vi "RT_SynthFoc_V2_GPU.vi"(0 "Ann Array Params":T1={"Synth Foc?"=FALSE, "Focal Zones"=41, "Switch T/R"=0, "Trans Geometry (mm)"={"Transducer"=0, "Geo Focus"=12.0, "a (radius)"=3.0, "# of rings"=5, "kerf space "=0.1, "Center Freq"=12.0}, "Sub Ap Excite?"=FALSE, "Full Array Scan?"=FALSE, "Xmt/Rcv"={"XMIT"=[TRUE, TRUE, TRUE, TRUE, TRUE], "RCV"=[TRUE, TRUE, TRUE, TRUE, TRUE]}, "PulseSpacing (us)"=0.0, "Xmit Ring"=0, "XMIT CHS"=0, "RCV CHS"=0, "GPU?"=FALSE, "Save TIFF?"=FALSE, "downfactor"=1, "RCV 1CH"=0} {"RCV 1CH" items=["All", "1", "2", "3", "4", "5"]; "Trans Geometry (mm)"."Transducer" items=["6D 12R 40 MHz"=0, "10D 31R 20 MHz"=1, "10D 23R 20 MHz"=2, "6D 23R 40 MHz"=3, "4.5D 10.7R 40 MHz"=4, "9D 23.5R 20 MHz"=5, "9D 25.8R 20MHz"=6, "Enter"=99]; "Switch T/R" min=1 max=5 step=1}, 2 "Pause?":bool, 3 "Motion Settings":T4={"No Motion?"=FALSE, "Motion System"=enum."NI 735x", "Motion Bd ID"=1, "Motion Profile"="SMAC1", "# Axis"=1, "Reverse Z axis?"=TRUE, "SMAC Axis"=0, "scan pair"=enum."y-(x) scan", "RT fps"=6.0, "Steps per mm"=[1000, 1000, 1000, 1000], "Motor Parameters"={"velocity ct/s"=[10000.0, 10000.0, 10000.0, 50000.0], "accel ct/s^2"=[50000.0, 50000.0, 50000.0, 200000.0]}, "One Way Scan"=FALSE, "Reverse One Way Scan"=FALSE, "Global Position (mm)"=[], "Plane"=0, "Distance between\nscan lines (um)"=0.0, "Distance between\nscan planes (um)"=0.0, "number of scan planes"=1, "Total steps in line"=0, "Xtra plane\ndistance  (um)"=100, "Xtra planes "=1, "Add Axis"=FALSE, "overshoot cts"=200, "BKPT Shift"=0, "Scan Start Time (ms)"=0, "ESP VISA"="GPIB::1::INSTR", "3rd Axis"=1, "GL Ref Out"=refnum, "Galil Address"=""} {"3rd Axis" items=["x", "y", "z", "w"]; "Xtra planes" min=1; "Xtra plane\ndistance  (um)" min=0; "Distance between\nscan planes (um)" format="%.2f"; "Distance between\nscan lines (um)" format="%.2f"; "SMAC Axis" items=["None"=0, "Axis 1"=1, "Axis 2"=2, "Axis 3"=3, "Axis 4"=4, "Axis 5"=5, "Axis 6"=6, "Axis 7"=7, "Axis 8"=8, "Vector Space 1"=17, "Vector Space 2"=18, "Vector Space 3"=19, "Vector Space 4"=20]; "Motion Bd ID" min=1 max=32 step=1}, 4 "Scan Axis":i32, 7 "Digitizer Settings":T8={"Digitizer delay (us) "=0.0, "rf points per line"=2048, "lines per plane"=128, "Samp Rate (Hz)"=100000000.0, "Additional dig delay (us)"=0.0, "Voltage Scale"=0.4, "Pre-Looks"=0, "Offset delay (us)"=0.0, "bits A/D"=8, "Avg Num"=1, "DigTimeOut"=5.0, "Rel Dig Delay"=0.0, "Dig Ch"=0, "LeCroyCluster"={"LeCroy Channels"=[TRUE, FALSE, FALSE, FALSE], "LC read pt offset"=0.0, "Sweep Avg"=FALSE}, "Main Digitizer"=enum."NI Digitizer", "Dig Config"=enum."Single channel", "Digitizer ID Cluster"={"Acqiris/Alazar/SP ID"=[], "NI Instr Handles"=[], "LeCroy VISA"="", "GaGe Handle"={"Handle"=0, "Sample size"=0, "Resolution"=0, "Offset"=0, "Channels"=0, "Boards"=0}, "ATS Ref"="ATS9350", "Acqiris Address"=["PCI::INSTR0"], "ADQRef"=refnum, "adq_cu_ptr"=refnum}, "Trigger Settings"={"Trig Source"=1, "Trig Coupling"=0, "Trig Slope"=0, "Level (mV)"=1500.0}, "Bulk Acq"=FALSE, "Bulk Start Indexes"=[], "Data Ref RF"=refnum, "NI ID/Channel"=[], "Total Dig CH"=1, "Xtra Ann Trig delay (us)"=10.0, "Fix Z Delay?"=FALSE, "One Way Transmission?"=FALSE, "Data Ref Log"=refnum} {"Trigger Settings"."Trig Slope" items=["Positive", "Negative"]; "Trigger Settings"."Level (mV)" format="%.2f"; "Trigger Settings"."Trig Coupling" items=["DC 1 MOhm", "AC 1 MOhm", "DC 50 Ohm", "AC 50 Ohm"]; "Trigger Settings"."Trig Source" items=["Chan 1", "External"]; "Rel Dig Delay" format="%.2f"; "DigTimeOut" format="%.2f"; "Avg Num" min=1; "Offset delay (us)" format="%.2f"; "Additional dig delay (us)" format="%.2f"; "Digitizer delay (us)" format="%.2f"}, 9 "Qs and Notis":T12, 11 "Raw Name":string="raw") -> (16 "Bd ID Out":u8, 19 "error out":errorcluster)   [LabVIEW 2022 SP3]
uses:
  <vilib>/picture/picture.llb/imagedata.ctl
  ScanningControl/Digitizers/-DigitizerRoutines/DigitizerSettings.ctl
  ScanningControl/Digitizers/-DigitizerRoutines/Digitizer.ctl
  ScanningControl/Digitizers/-DigitizerRoutines/DigConfig.ctl
  ScanningControl/Digitizers/-DigitizerRoutines/DigitizerID.ctl
  C:/Windows/System32/ADQAPI_dotNet_helper.dll
  Windows/System32/ADQAPI_dotNet_helper.dll
  ScanningControl/Motion Controllers/NI_controller/-NI_MotionRoutines/MotionParameters.ctl
  ScanningControl/Motion Controllers/NI_controller/-NI_MotionRoutines/MotionSys.ctl
  ScanningControl/Motion Controllers/-MotionRoutines/ScanAxis.ctl
  ScanningControl/Motion Controllers/-MotionRoutines/3rdAxis.ctl
  Annular Array/-AnnularRoutines/AnnularArray.ctl
  Annular Array/-AnnularRoutines/TransGeometry.ctl
  Annular Array/-AnnularRoutines/ArrayGeometry.ctl
  ScanningControl/Motion Controllers/Galil/Command Menu.ctl
  <vilib>/DAQmx/write.llb/DAQmx Write (Digital Bool 1Line 1Point).vi
  <instrlib>/niScope/Acquire/niScope Get Scaling Coefficients.vi
  ScanningControl/Motion Controllers/-MotionRoutines/MotionGlobals.vi
  <vilib>/DAQmx/miscellaneous.llb/DAQmx Fill In Error Info.vi
  <instrlib>/niScope/Acquire/Fetch/niScope Multi Fetch Binary 8.vi
  <vilib>/Motion/FlexMotion/FunctionsVIs/Trajectory.llb/Load Acceleration/Deceleration.flx
  <vilib>/Motion/FlexMotion/CustomControls/CustomControls.llb/Program.flx
  <vilib>/Motion/FlexMotion/FunctionsVIs/Trajectory.llb/Wait for Move Complete (8 axes).flx
  <vilib>/Analysis/NI_AALPro.lvlib
  <instrlib>/LeCroy Wave Series/LeCroy Wave Series.lvlib
panel:
  in  "Round to ROC?":bool
  in  "One Way Receive":bool
  # "1-D and 2-D B scan settings"
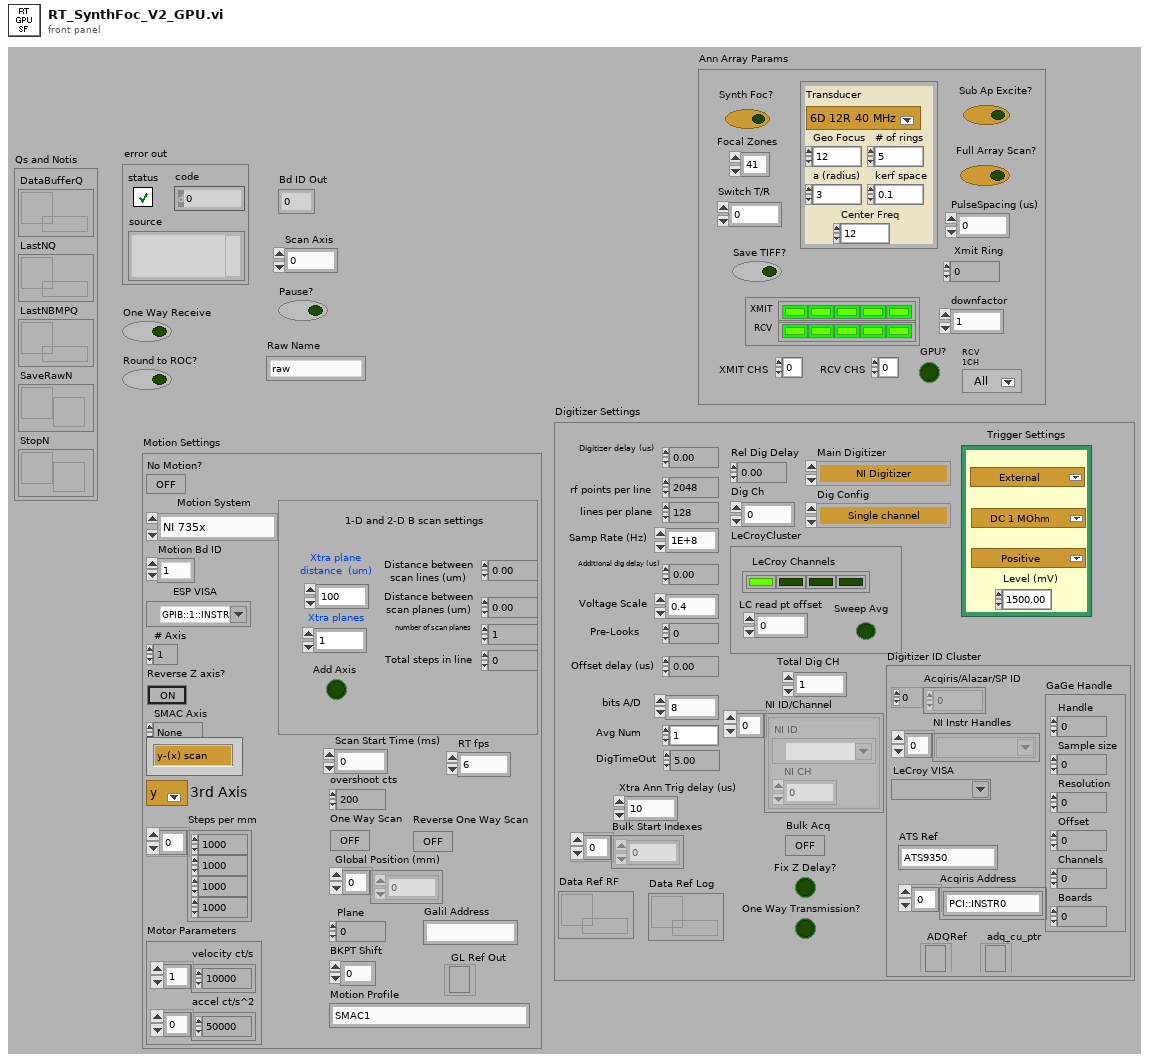
[diagram p1: front panel]
types:
  T1 = typedef "AnnularArray.ctl" = cluster{"Synth Foc?":bool, "Focal Zones":i16, "Switch T/R":i16, "Trans Geometry (mm)":T2, "Sub Ap Excite?":bool, "Full Array Scan?":bool, "Xmt/Rcv":cluster{"XMIT":bool[], "RCV":bool[]}, "PulseSpacing (us)":sgl, "Xmit Ring":i32, "XMIT CHS":u8, "RCV CHS":u8, "GPU?":bool, "Save TIFF?":bool, "downfactor":i32, "RCV 1CH":u16}
  T2 = typedef "TransGeometry.ctl" = cluster{"Transducer":T3, "Geo Focus":dbl, "a (radius)":dbl, "# of rings":i32, "kerf space ":dbl, "Center Freq":dbl}
  T3 = typedef "ArrayGeometry.ctl" = u16
  T4 = typedef "MotionParameters.ctl" = cluster{"No Motion?":bool, "Motion System":T5, "Motion Bd ID":u8, "Motion Profile":string, "# Axis":i8, "Reverse Z axis?":bool, "SMAC Axis":u16, "scan pair":T6, "RT fps":sgl, "Steps per mm":i32[], "Motor Parameters":cluster{"velocity ct/s":dbl[], "accel ct/s^2":dbl[]}, "One Way Scan":bool, "Reverse One Way Scan":bool, "Global Position (mm)":dbl[], "Plane":i32, "Distance between\nscan lines (um)":sgl, "Distance between\nscan planes (um)":sgl, "number of scan planes":i32, "Total steps in line":i32, "Xtra plane\ndistance  (um)":i32, "Xtra planes ":i32, "Add Axis":bool, "overshoot cts":i32, "BKPT Shift":i32, "Scan Start Time (ms)":u32, "ESP VISA":refnum<visa-resource-name>, "3rd Axis":T7, "GL Ref Out":refnum<k7>, "Galil Address":string}
  T5 = typedef "MotionSys.ctl" = enum16{"MM3000", "NI 735x", "Newport ESP", "No Motion Card", "Galil"}
  T6 = typedef "ScanAxis.ctl" = enum16{"y-(x) scan", "x-(y) scan", "z-(x) scan", "z-(y) scan", "y-(z) scan", "x-(z) scan", "w-(x) scan", "w-(y) scan", "w-(z) scan", "x-(w) scan", "y-(w) scan", "z-(w) scan"}
  T7 = typedef "3rdAxis.ctl" = u16
  T8 = typedef "DigitizerSettings.ctl" = cluster{"Digitizer delay (us) ":dbl, "rf points per line":i32, "lines per plane":i32, "Samp Rate (Hz)":dbl, "Additional dig delay (us)":dbl, "Voltage Scale":dbl, "Pre-Looks":i32, "Offset delay (us)":dbl, "bits A/D":i8, "Avg Num":i32, "DigTimeOut":sgl, "Rel Dig Delay":sgl, "Dig Ch":i32, "LeCroyCluster":cluster{"LeCroy Channels":bool[], "LC read pt offset":dbl, "Sweep Avg":bool}, "Main Digitizer":T9, "Dig Config":T10, "Digitizer ID Cluster":T11, "Trigger Settings":cluster{"Trig Source":u16, "Trig Coupling":u16, "Trig Slope":u16, "Level (mV)":dbl}, "Bulk Acq":bool, "Bulk Start Indexes":i32[], "Data Ref RF":refnum<data-value>, "NI ID/Channel":cluster{"NI ID":refnum<k15>, "NI CH":i32}[], "Total Dig CH":i32, "Xtra Ann Trig delay (us)":dbl, "Fix Z Delay?":bool, "One Way Transmission?":bool, "Data Ref Log":refnum<data-value>}
  T9 = typedef "Digitizer.ctl" = enum16{"Acqiris Digitizer", "NI Digitizer", "LeCroy", "GaGe", "AlazarTech", "No Digitizer", "Teledyne"}
  T10 = typedef "DigConfig.ctl" = enum16{"Single channel", "2 Chans w/ 2 Acqiris", "2 Chans w/ 1 Acqiris", "5-CH Pulser New", "5-CH pulser w/ ann array", "5-pass style ann array", "Empty"}
  T11 = typedef "DigitizerID.ctl" = cluster{"Acqiris/Alazar/SP ID":u32[], "NI Instr Handles":refnum<k15>[], "LeCroy VISA":refnum<visa-resource-name>, "GaGe Handle":cluster{"Handle":u32, "Sample size":u32, "Resolution":i32, "Offset":i32, "Channels":u32, "Boards":u32}, "ATS Ref":string, "Acqiris Address":string[], "ADQRef":refnum<k24>, "adq_cu_ptr":refnum<k24>}
  T12 = cluster{"DataBufferQ":refnum<queue>, "LastNQ":refnum<queue>, "LastNBMPQ":refnum<queue>, "SaveRawN":refnum<notifier>, "StopN":refnum<notifier>}
  T13 = cluster{"offset":dbl, "gain":dbl, "reserved 1":dbl, "reserved 2":dbl}[]
  T14 = cluster{"offset":dbl, "gain":dbl, "reserved 1":dbl, "reserved 2":dbl}
  T15 = cluster{sgl, "Gain [dB]  ":sgl, "Atten (dB)":sgl}
  T16 = typedef "location.ctl" = enum16{"Automatic", "WCM Main", "Hawaii", "Columbia MM3000", "Columbia  NI System", "NYU", "RRI 2", "UHI Allen", "CUMC RT", "Chiba", "Stony Brook", "WCM Microscopy", "WCM Aeoretch", "WCM Optics Lab", "WCM Main 2Axis", "WCM Rotation", "WCM SAM SMAC", "SERI GP"}
  T17 = typedef "Command Menu.ctl" = enum16{"CommandPassThrough", "Abort Motion", "Define Pos", "Velocity", "Acceleration", "Deceleration", "Position Rel", "Postion Abs", "Begin Move", "After Move", "Home", "KI", "KD", "KP", "IL", "Config I/O", "Set Bit", "Clear Bit", "Motor Off", "Moto On", "Status", "Execute", "Halt Execute", "HX Status", "Tell Velocity", "Check Motion", "BreakPoint", "Tell Position", "Current Code Line", "Tell Switches", "OC Force On", "OC Off", "Pos Soft Limit", "Rev Soft Limit"}
  T18 = cluster{"gain":dbl, "wfm":i16[], bool, bool, i32}
  T19 = typedef "Program.flx" = u8
  T20 = cluster{"data value reference":refnum<data-value>, "bytes to transfer":u32, "rf pts actual":u32}
  T21 = cluster{"gain":dbl, bool, "RF_Out":i16[][], "count":i32, bool}
  T22 = cluster{"actualSamples":i32, "absoluteInitialX":dbl, "relativeInitialX":dbl, "xIncrement":dbl, "offset":dbl, "gain":dbl, "reserved1":dbl, "reserved2":dbl}[]
  T23 = cluster{"actualSamples":i32, "absoluteInitialX":dbl, "relativeInitialX":dbl, "xIncrement":dbl, "offset":dbl, "gain":dbl, "reserved1":dbl, "reserved2":dbl}
  T24 = cluster{"gain":dbl, "Sorted Array Out":i16[], "Reverse?":bool, "status":bool, i32}
  T25 = cluster{"Raw VGain (scale)":dbl, "Sorted Array Out":i16[], "Reverse?":bool, "status":bool, i32}
  T26 = cluster{"Voltage Scale":dbl, "DataInterleavedOut":i16[], "Reverse?":bool, bool, i32}
  T27 = typedef "Bd Id Out" = u8
  T28 = typedef "Resource Out (Enum).flx" = u16
  T29 = typedef "GL Axis Control.ctl" = u16
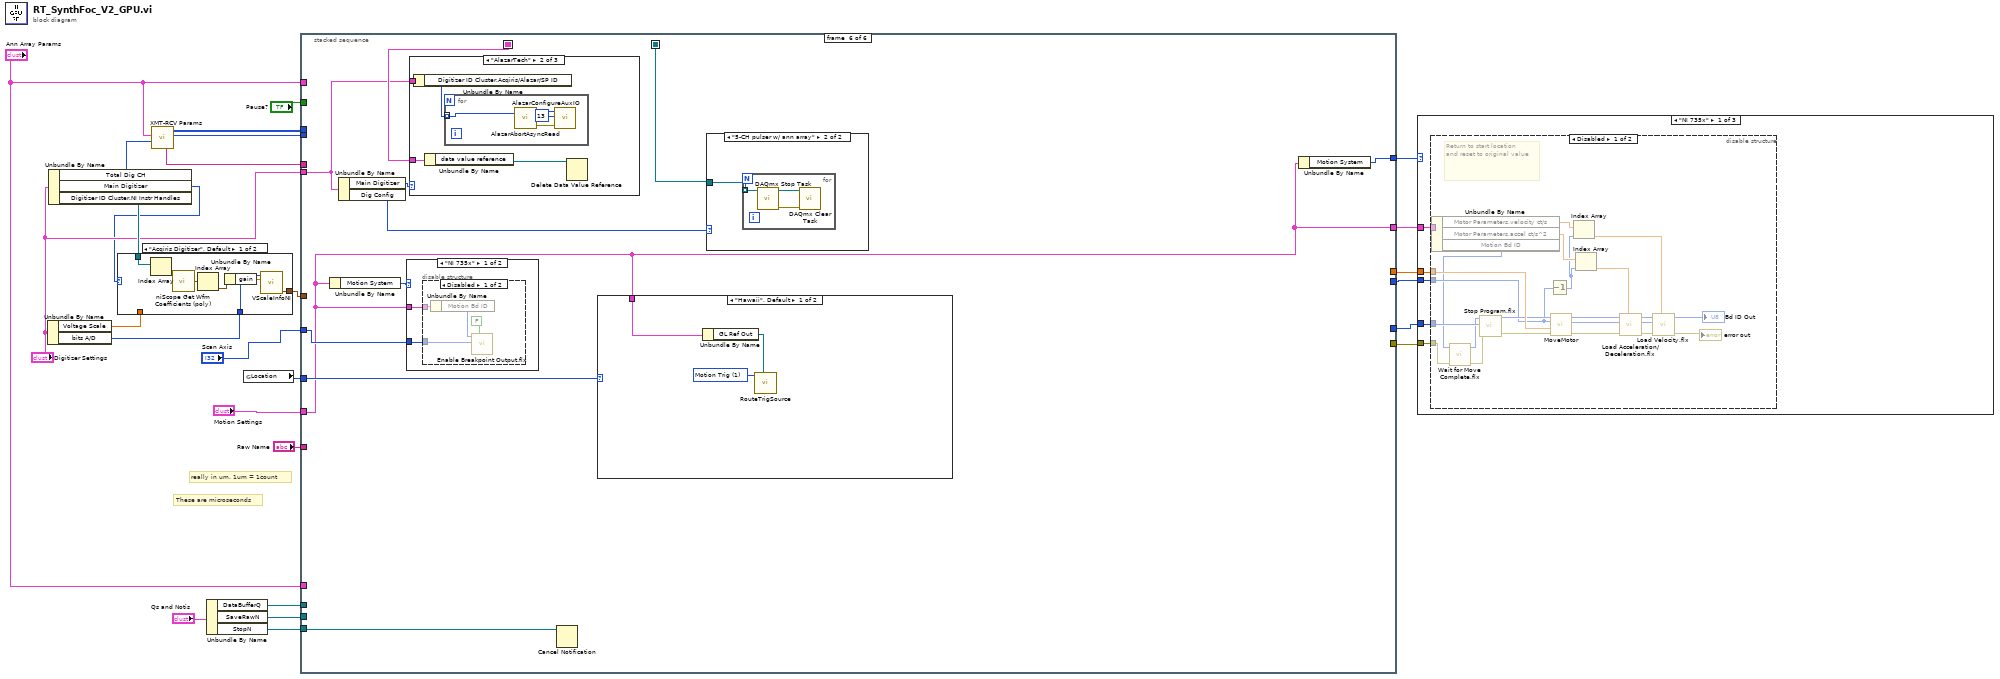
[diagram p0: block diagram]
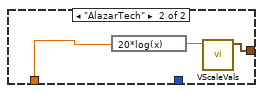
[diagram p2: hidden frame]
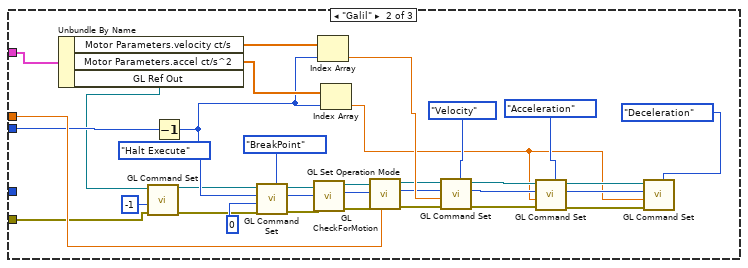
[diagram p4: hidden frame]
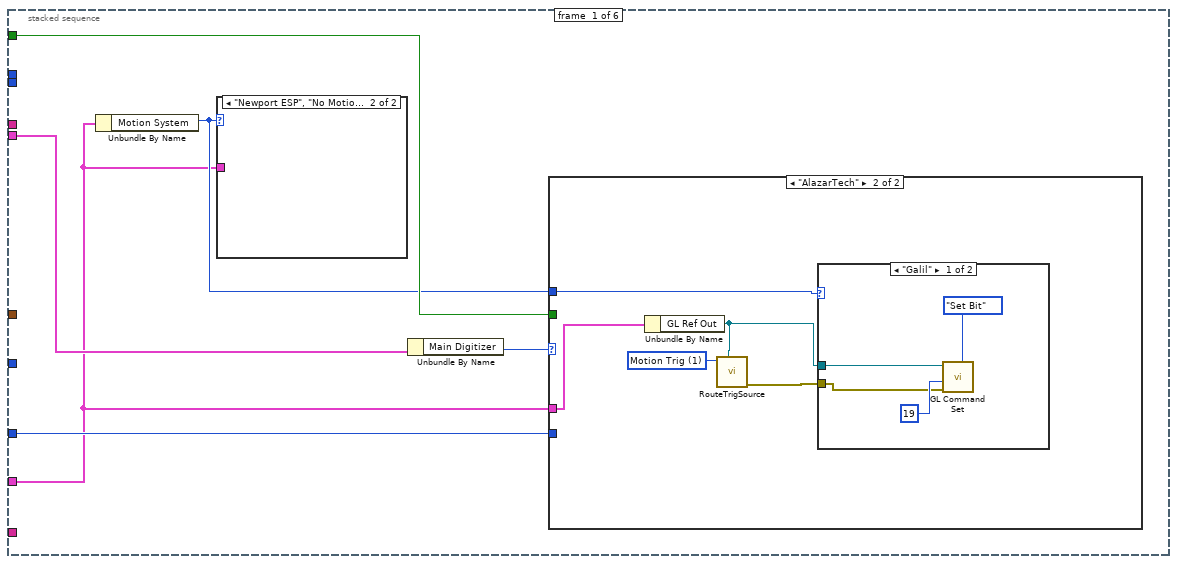
[diagram p6: hidden frame]
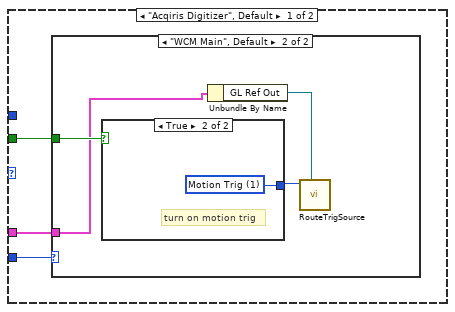
[diagram p7: hidden frame]
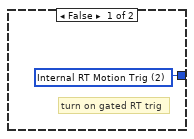
[diagram p9: hidden frame]
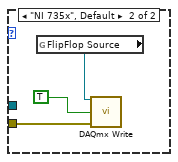
[diagram p10: hidden frame]
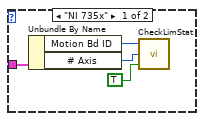
[diagram p11: hidden frame]
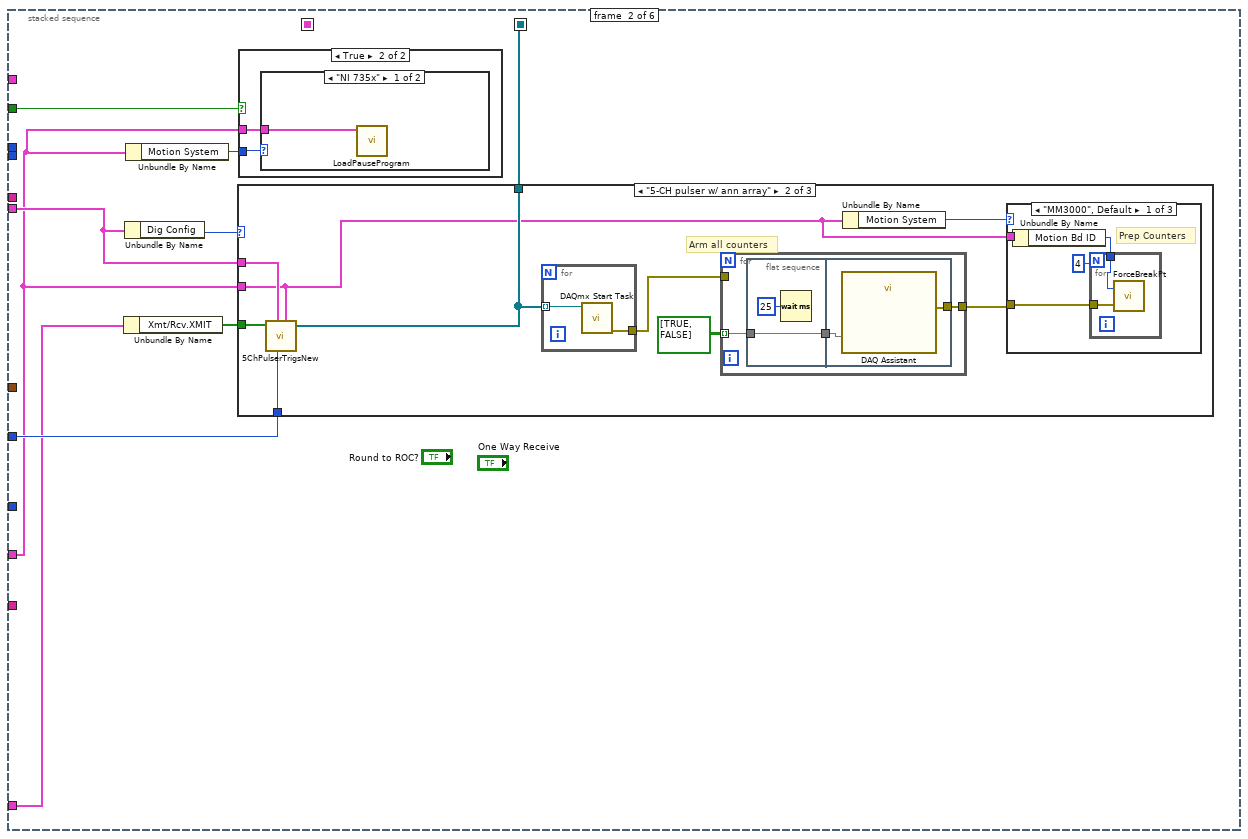
[diagram p12: hidden frame]
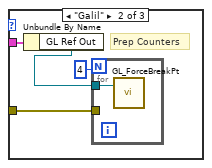
[diagram p14: hidden frame]
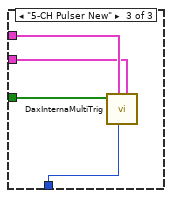
[diagram p16: hidden frame]
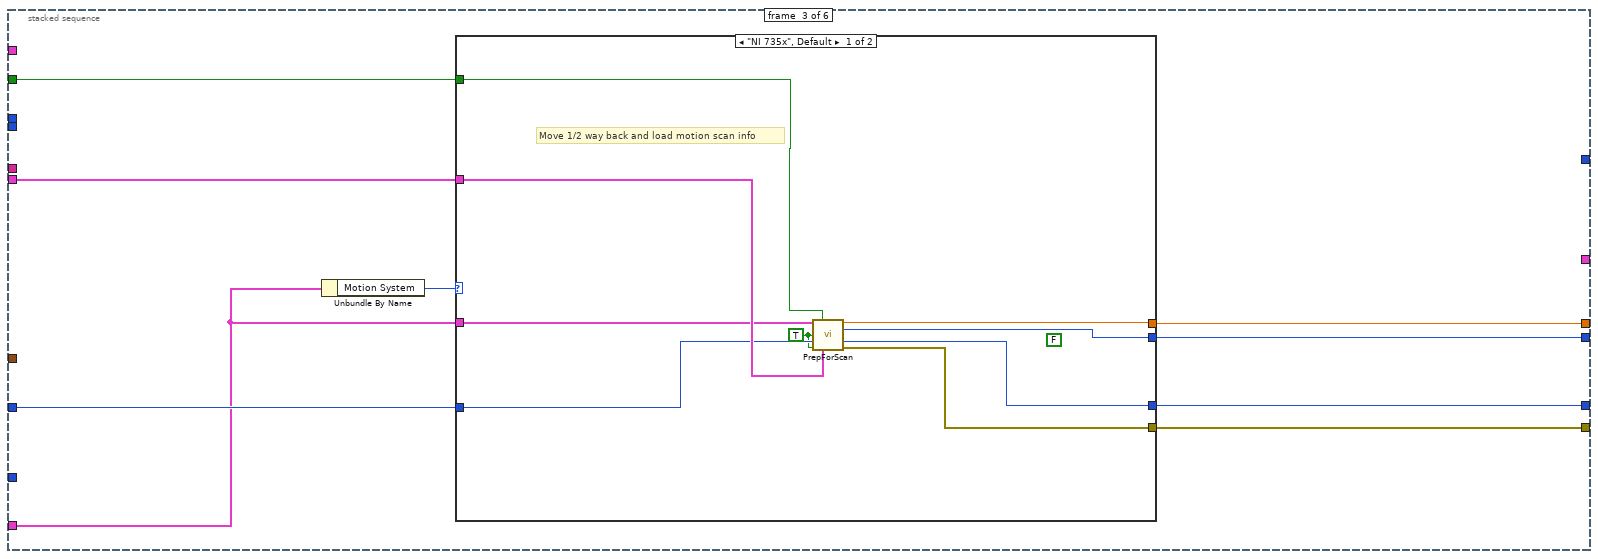
[diagram p19: hidden frame]
diagram:
  # "These are microseconds"
  # "really in um. 1um = 1count"
  n1 = Unbundle By Name("Digitizer Settings") -> ("Voltage Scale"=w11:dbl, "bits A/D"=w10:i8)
  n2 = Unbundle By Name("Digitizer Settings") -> ("Total Dig CH"=w2:i32, "Main Digitizer"=w8:T9, "Digitizer ID Cluster.NI Instr Handles"=w12:refnum<k15>[])
  n3 = case shown="\"Acqiris Digitizer\", Default" w8 {
    tunnel: [w29 w35] -> w15
    tunnel: w12 -> [w28 _]
    tunnel: w10 -> [w27 _]
    tunnel: w11 -> [_ w34]
    frame "Acqiris Digitizer", Default {
      n4 = Index Array(array=w28) -> (element=w31:refnum<k15>)  [unwired: 1 in]
      n5 = call-poly <instrlib>:"niScope Get Wfm Coefficients (poly).vi"("instrument handle"=w31) -> ("coefficient info"=w32:T13)  [unwired: 12 in, 2 out]
      n6 = Index Array(array=w32) -> (element=w33:T14)  [unwired: 1 in]
      n7 = Unbundle By Name(w33) -> ("gain"=w30:dbl)
      n8 = call "VScaleInfoNI.vi"("A/D bits"=w27, "gain"=w30) -> ("Voltage Scale"=w29:T15)  [unwired: 5 in, 3 out]
    }
    frame "AlazarTech" {
      n9 = expression code="20*log(x)"(w34) -> (w36:dbl)
      n10 = call "VScaleVals.vi"("Full Scale"=w36) -> ("Voltage Scale"=w35:T15)  [unwired: 8 in, 2 out]
    }
  }
  n11 = call "XMT-RCV Params.vi"("Dig Channels"=w2, "Ann Array Params"="Ann Array Params") -> ("# XMIT"=w14:i16, "Recip Table"=w13:i16[][], "T/R String"=w7:string)  [unwired: 4 in, 3 out]
  n12 = Unbundle By Name("Qs and Notis") -> ("DataBufferQ"=w20:refnum<queue>, "SaveRawN"=w19:refnum<notifier>, "StopN"=w21:refnum<notifier>)
  n13 = global read "MotionGlobals.vi" "Location"() -> (w16:T16)
  n14 = stacked-sequence {
    seq-local: [_ w75 _ _ _ _] -> [_ _ _ _ _ w552]
    seq-local: [_ _ _ w135 _ _] -> [_ _ _ _ w192 w548]
    tunnel: [_ _ w121 _ _ _] -> w24
    tunnel: [_ _ w120 _ _ _] -> w25
    tunnel: [_ _ w117 _ _ _] -> w23
    tunnel: [_ _ w119 _ _ _] -> w26
    tunnel: "Scan Axis" -> [_ w74 w118 _ _ w549]
    tunnel: w21 -> [_ _ _ _ w216 w550]
    tunnel: w20 -> [_ _ _ _ w205 _]
    tunnel: w16 -> [w42 _ _ _ _ w551]
    tunnel: "Pause?" -> [w41 w76 w116 _ w215 _]
    tunnel: w19 -> [_ _ _ _ w214 _]
    tunnel: "Raw Name" -> [_ _ _ _ w213 _]
    tunnel: w15 -> [_ _ _ _ w211 _]
    tunnel: w14 -> [_ _ _ w137 w210 _]
    tunnel: w13 -> [_ _ _ _ w188 _]
    tunnel: w7 -> [_ _ _ _ w209 _]
    tunnel: "Digitizer Settings" -> [w39 w72 w115 w132 w185 w547]
    tunnel: "Motion Settings" -> [w37 w68 w114 _ w197 w542]
    tunnel: [_ _ _ _ _ w543] -> w6
    tunnel: [_ _ _ _ _ w542] -> w5
    tunnel: "Ann Array Params" -> [_ w69 _ _ w183 _]
    tunnel: "Ann Array Params" -> [_ _ _ _ w187 _]
    frame #0 {
      n15 = Unbundle By Name(w37) -> ("Motion System"=w38:T5)
      n16 = case shown="\"Newport ESP\", \"No Motion Card\", Default" w38 {
        tunnel: w37 -> [w67 _]
        frame "NI 735x" {
          n17 = Unbundle By Name(w67) -> ("Motion Bd ID"=w66:u8, "# Axis"=w65:i8)
          n18 = call "CheckLimStat.vi"("Always Warn?"=TRUE, "# Axis"=w65, "Motion Board ID"=w66) -> ()  [unwired: 3 in]
        }
        frame "Newport ESP", "No Motion Card", Default {
        }
      }
      n19 = Unbundle By Name(w39) -> ("Main Digitizer"=w40:T9)
      n20 = case shown="\"AlazarTech\"" w40 {
        tunnel: w42 -> [w45 _]
        tunnel: w41 -> [w44 _]
        tunnel: w38 -> [_ w54]
        tunnel: w37 -> [w43 w53]
        frame "Acqiris Digitizer", Default {
          n21 = case shown="\"WCM Main\", Default" w45 {
            tunnel: w44 -> [_ w49]
            tunnel: w43 -> [_ w47]
            frame "UHI Allen", "CUMC RT" {
            }
            frame "WCM Main", Default {
              n22 = case shown="True" w49 {
                tunnel: [w50 w51] -> w48
                frame False {
                  w50 = u16 2 items=["Function Gen Input", "Motion Trig", "Internal RT Motion Trig", "Internal CTR 1 Output"] ("Trig Source")
                  # "turn on gated RT trig"
                }
                frame True {
                  w51 = u16 1 items=["Function Gen Input", "Motion Trig", "Internal RT Motion Trig", "Internal CTR 1 Output"] ("Trig Source")
                  # "turn on motion trig"
                }
              }
              n23 = Unbundle By Name(w47) -> ("GL Ref Out"=w46:refnum<k7>)
              n24 = call "RouteTrigSource.vi"("Galil.IGalil"=w46, "Trig Source"=w48) -> ()  [unwired: 9 in, 1 out]
            }
          }
        }
        frame "AlazarTech" {
          w56 = u16 1 items=["Function Gen Input", "Motion Trig", "Internal RT Motion Trig", "Internal CTR 1 Output"] ("Trig Source")
          n25 = Unbundle By Name(w53) -> ("GL Ref Out"=w52:refnum<k7>)
          n26 = call "RouteTrigSource.vi"("Galil.IGalil"=w52, "Trig Source"=w56) -> ("error out"=w55:errorcluster)  [unwired: 9 in]
          n27 = case shown="\"Galil\"" w54 {
            tunnel: w55 -> [w58 w61]
            tunnel: w52 -> [w57 _]
            frame "Galil" {
              n28 = call "GL Command Set.vi"("Command"=Command_Menu."Set Bit", "error in (no error)"=w58, "Value"=19, "Galil.IGalil"=w57) -> ()  [unwired: 3 in, 5 out]
            }
            frame "NI 735x", Default {
              n29 = global read "MotionGlobals.vi" "FlipFlop Source"() -> (w62:refnum<k21>)
              n30 = call-poly <vilib>:"DAQmx Write.vi"("task/channels in"=w62, "data"=TRUE ("stop (T)"), "error in"=w61) -> ()  [unwired: 10 in, 3 out]
            }
          }
        }
      }
    }
    frame #1 {
      n31 = Unbundle By Name(w69) -> ("Xmt/Rcv.XMIT"=w70:bool[])
      n32 = Unbundle By Name(w72) -> ("Dig Config"=w73:T10)
      n33 = Unbundle By Name(w68) -> ("Motion System"=w71:T5)
      n34 = case shown="\"5-CH pulser w/ ann array\"" w73 {
        tunnel: w74 -> [_ w85 w106]
        tunnel: [_ w84 _] -> w75
        tunnel: w70 -> [_ w80 w107]
        tunnel: w72 -> [_ w79 w109]
        tunnel: w68 -> [_ w77 w108]
        frame "Single channel", Default {
        }
        frame "5-CH pulser w/ ann array" {
          # "Arm all counters"
          n35 = call "5ChPulserTrigsNew.vi"("Motion Settings"=w77, "Digitizer Settings"=w79, "XMIT"=w80, "Axis"=w85) -> ("5CH Pulser Tasks"=w84:refnum<k21>[])  [unwired: 5 in, 1 out]
          n36 = for {
            tunnel: w84 -> [w98] mode=indexing
            tunnel: [w97] -> w82
            n37 = call <vilib>:"DAQmx Start Task.vi"("task/channels in"=w98) -> ("error out"=w97:errorcluster)  [unwired: 1 in, 13 out]
          }
          n38 = for {
            tunnel: bool[][] [[TRUE], [FALSE]] ("data") -> [w100] mode=indexing
            tunnel: w82 -> [_]
            tunnel: [w99] -> w81
            n39 = flat-sequence {
              tunnel: w100 -> [w103]
              tunnel: [w103] -> w101
              tunnel: w101 -> [w105]
              tunnel: [w104] -> w99
              frame #0 {
                n40 = Wait (ms)(milliseconds to wait=u32 25) -> ()  [unwired: 1 out]
              }
              frame #1 {
                n41 = call "DAQ Assistant"("data"=w105) -> ("error out"=w104:errorcluster)  [unwired: 17 in, 1 out]
              }
            }
          }
          n42 = Unbundle By Name(w77) -> ("Motion System"=w78:T5)
          n43 = case shown="\"MM3000\", Default" w78 {
            tunnel: w81 -> [w88 w94 _]
            tunnel: w77 -> [w86 w93 _]
            frame "MM3000", Default {
              # "Prep Counters"
              n44 = Unbundle By Name(w86) -> ("Motion Bd ID"=w87:u8)
              n45 = for {
                N: 4 -> [_]
                tunnel: w88 -> [w91]
                tunnel: w87 -> [w90]
                n46 = call "ForceBreakPt.vi"("error in"=w91, "Bd ID in"=w90) -> ()  [unwired: 2 out]
              }
            }
            frame "Galil" {
              # "Prep Counters"
              n47 = Unbundle By Name(w93) -> ("GL Ref Out"=w92:refnum<k7>)
              n48 = for {
                N: 4 -> [_]
                tunnel: w94 -> [_]
                tunnel: w92 -> [w96]
                n49 = call "GL_ForceBreakPt.vi"("GL Ref Out"=w96) -> ()  [unwired: 1 in, 2 out]
              }
            }
            frame "No Motion Card" {
            }
          }
        }
        frame "5-CH Pulser New" {
          n50 = call "DaxInternaMultiTrig.vi"("Motion Settings"=w108, "Digitizer Settings"=w109, "XMIT"=w107, "Axis"=w106) -> ()  [unwired: 6 in, 1 out]
        }
      }
      n51 = case shown="True" w76 {
        tunnel: w71 -> [_ w111]
        tunnel: w68 -> [_ w110]
        frame False {
        }
        frame True {
          n52 = case shown="\"NI 735x\"" w111 {
            tunnel: w110 -> [w112 _]
            frame "NI 735x" {
              n53 = call "LoadPauseProgram.vi"("Motion Settings"=w112) -> ()  [unwired: 10 in, 1 out]
            }
            frame "No Motion Card", Default {
            }
          }
        }
      }
    }
    frame #2 {
      n54 = Unbundle By Name(w114) -> ("Motion System"=w113:T5)
      n55 = case shown="\"NI 735x\", Default" w113 {
        tunnel: [w127 _] -> w121
        tunnel: [w126 _] -> w120
        tunnel: [w125 _] -> w119
        tunnel: w118 -> [w129 _]
        tunnel: [w128 _] -> w117
        tunnel: w116 -> [w123 _]
        tunnel: w115 -> [w130 _]
        tunnel: w114 -> [w122 _]
        frame "NI 735x", Default {
          w124 = TRUE ("Boolean")
          (unwired) FALSE ("Enable")
          # "Move 1/2 way back and load motion scan info"
          n56 = call "PrepForScan.vi"("Motion Settings In"=w122, "Pause?"=w123, "SMAC?"=w124, "Scan Axis"=w129, "MoveBack?"=w124, "Digitizer Settings"=w130) -> ("Counts"=w128:dbl, "Axis Resource out"=w125:u16, "Program ID"=w126:u8, "error out"=w127:errorcluster)  [unwired: 4 in, 2 out]
        }
        frame "No Motion Card" {
        }
      }
    }
    frame #3 {
      # "Set up sampling rete and delay"
      n57 = Unbundle By Name(w132) -> ("Main Digitizer"=w131:T9, "lines per plane"=w133:i32, "rf points per line"=w134:i32)
      n58 = Multiply(x=w137, y=w133) -> (x*y=w136:i32)
      n59 = case shown="\"AlazarTech\"" w131 {
        tunnel: w134 -> [w141 w154 _]
        tunnel: w136 -> [w140 w153 w169]
        tunnel: [_ w155 _] -> w135
        tunnel: w132 -> [w138 w156 w170]
        frame "Acqiris Digitizer", Default {
          n60 = Unbundle By Name(w138) -> ("Digitizer ID Cluster.NI Instr Handles"=w139:refnum<k15>[])
          n61 = for {
            tunnel: w140 -> [w144]
            tunnel: w141 -> [w148]
            tunnel: w139 -> [w145] mode=indexing
            tunnel: w138 -> [w142]
            n62 = property class="niScope"(reference=w145, "Min Number of Points"=w148, "Number of Records"=w144, "Enable Records > Memory"=TRUE) -> (reference out=w147:refnum<k15>, error out=w146:errorcluster)  [unwired: 1 in]
            n63 = call "NI conSamp.vi"("error in"=w146, "Digitizer Settings"=w142, "InstrumentID"=w147) -> ()  [unwired: 1 in, 2 out]
          }
        }
        frame "AlazarTech" {
          n64 = Unbundle By Name(w156) -> ("Digitizer ID Cluster.GaGe Handle.Boards"=w149:u32, "Digitizer ID Cluster.Acqiris/Alazar/SP ID"=w151:u32[])
          n65 = case shown="2, Default" w149 {
            tunnel: [w158 w159] -> w152
            frame 2, Default {
              w158 = u32 3 items=["A"=1, "B"=2, "A + B"=3, "C"=4, "A + C"=5, "A + B"=6, "D"=8, "A + D"=9, "B + D"=10, "C + D"=12, "A + B + C + D"=15] ("Channel")
            }
            frame 16 {
              w159 = u32 15 items=["A"=1, "B"=2, "A + B"=3, "C"=4, "A + C"=5, "A + B"=6, "D"=8, "A + D"=9, "B + D"=10, "C + D"=12, "A + B + C + D"=15] ("Channel")
            }
          }
          n66 = for {
            tunnel: w152 -> [w168]
            tunnel: [w165] -> w157
            tunnel: w156 -> [w164]
            tunnel: [w163] -> w155
            tunnel: w154 -> [w162]
            tunnel: w153 -> [w161]
            tunnel: w151 -> [w160] mode=indexing
            n67 = call "AlazarAcqPrep - ATS-SDK.vi"("Handle"=w160, "Digitizer Settings"=w164, "Enable Trigger Enable"=TRUE, "Channel"=w168, "BuffCount"=6, "rf points per line"=w162, "rf lines per buffer"=w161) -> ("AlazarCluster"=w163:T20, "error out"=w165:errorcluster)  [unwired: 5 in, 2 out]
          }
          n68 = Index Array(array=w151) -> (element=w150:u32)  [unwired: 1 in]
          n69 = call "AlazarStartCapture.vi"("Handle"=w150, "error in (no error)"=w157) -> ()  [unwired: 3 out]
        }
        frame "LeCroy" {
          w180 = FALSE ("Continuous Acquisition Mode (T: On)")
          w171 = u16 2 items=["RealTime", "RIS", "Sequence", "Roll", "WaveStream"] ("Sample Mode (0: RealTime)")
          n70 = Unbundle By Name(w170) -> ("Digitizer ID Cluster.LeCroy VISA"=w173:refnum<visa-resource-name>, "Digitizer delay (us)"=w172:dbl)
          n71 = call <instrlib>:"Configure Continuous Acquisition.vi"("Auto Trigger Enabled (T: Normal)"=w180, "Continuous Acquisition Mode (T: On)"=w180, "VISA resource name"=w173) -> ("error out"=w181:errorcluster, "VISA resource name out"=w182:refnum<visa-resource-name>)  [unwired: 7 in]
          n72 = expression code="-1E-6*x"(w172) -> (w178:dbl)
          n73 = call <instrlib>:"Configure Sample Mode.vi"("error in (no error)"=w181, "Number of Segments (2)"=w169, "Sample Mode (0: RealTime)"=w171, "VISA resource name"=w182) -> ("error out"=w176:errorcluster, "VISA resource name out"=w177:refnum<visa-resource-name>)  [unwired: 6 in]
          n74 = Number To Exponential String(number=w178) -> (E-format string=w179:string)  [unwired: 3 in]
          n75 = Concatenate Strings("TRDL " ("Write Buffer"), w179) -> (w175:string)
          n76 = call <instrlib>:"Write.vi"("error in (no error)"=w176, "Write Buffer"=w175, "VISA resource name"=w177) -> ()  [unwired: 6 in, 3 out]
        }
      }
    }
    frame #4 {
      n77 = Unbundle By Name(w185) -> ("bits A/D"=w199:i8, "lines per plane"=w200:i32, "rf points per line"=w201:i32)
      n78 = Unbundle By Name(w185) -> ("Total Dig CH"=w196:i32)
      n79 = Multiply(x=w196, y=3) -> (x*y=w195:i32)
      n80 = Unbundle By Name(w192) -> ("rf pts actual"=w191:u32)
      n81 = Multiply(x=w210, y=w200) -> (x*y=w190:i32)
      n82 = Unbundle By Name(w187) -> ("Xmt/Rcv.RCV"=w186:bool[])
      n83 = call "RTHeader.vi"("Comment"=w209, "Digitizer Settings"=w185, "Dig Word Size"=w199, "Ann Array Params"=w183, "Votage scaling"=w211, "Motion Settings"=w197) -> ("Header String Out"=w207:string)  [unwired: 8 in, 1 out]
      n84 = Obtain Queue(max queue size (-1, unlimited)=w195, element data type=T18 {"gain"=0.0, "wfm"=[], TRUE, TRUE, 0}) -> (queue out=w206:refnum<queue>)  [unwired: 3 in, 2 out]
      n85 = Unbundle By Name(w185) -> ("Main Digitizer"=w198:T9)
      n86 = case shown="14" w199 {
        tunnel: [_ u16 3 ("Extra Shift")] -> w202
        frame 0, Default {
        }
        frame 14 {
        }
      }
      n87 = Initialize Array(i16 0, w190, w191) -> (w189:i16[][])
      n88 = Subtract(x=w199, y=w202) -> (x-y=w203:u16)
      n89 = while {
        tunnel: w206 -> [w243]
        tunnel: w201 -> [w242]
        tunnel: [w237] -> w204
        tunnel: w200 -> [w241]
        tunnel: w205 -> [w240]
        tunnel: w207 -> [w239]
        tunnel: w216 -> [w229]
        tunnel: w214 -> [w235]
        tunnel: w213 -> [w234]
        tunnel: w210 -> [w232]
        tunnel: w188 -> [w231]
        tunnel: w203 -> [w230]
        tunnel: w183 -> [w228]
        tunnel: w185 -> [w227]
        tunnel: 1000 ("timeout in ms (-1)") -> [w218]
        i -> [w233]
        stop <- w237 stop-if-true
        n90 = Dequeue Element(queue=w243, timeout in ms (-1)=w218) -> (element=w222:T18)  [unwired: 1 in, 3 out]
        n91 = Unbundle(w222) -> (w219:bool)  [unwired: 4 out]
        n92 = case shown="False" w219 {
          tunnel: w241 -> [_ _]
          tunnel: w242 -> [_ _]
          tunnel: [w263 _] -> w221
          tunnel: w239 -> [w262 _]
          tunnel: w222 -> [w261 _]
          tunnel: w235 -> [w259 _]
          tunnel: w234 -> [w258 _]
          tunnel: w233 -> [w257 _]
          tunnel: [w256 _] -> w220
          tunnel: w232 -> [_ _]
          tunnel: w231 -> [_ _]
          tunnel: w230 -> [w255 _]
          tunnel: w228 -> [w254 _]
          tunnel: w227 -> [w249 _]
          tunnel: [w246 _] -> w226
          tunnel: [w245 _] -> w224
          frame False {
            n93 = Unbundle(w261) -> ("gain"=w263:dbl, "wfm"=w253:i16[], w256:bool, w244:i32)  [unwired: 1 out]
            n94 = Get Notifier Status(notifier=w259) -> (current notification=w260:bool)  [unwired: 1 in, 4 out]
            n95 = Unbundle By Name(w249) -> ("bits A/D"=w248:i8)
            n96 = case shown="True" w260 {
              tunnel: w253 -> [_ w269]
              tunnel: w262 -> [_ w273]
              tunnel: w258 -> [_ w272]
              tunnel: w257 -> [_ w271]
              tunnel: w256 -> [_ _]
              tunnel: w255 -> [_ w270]
              frame False {
              }
              frame True {
                n97 = Build Array(w269) -> (w268:i16[][])
                n98 = call "RawRT_Capture.vi"("A/D bits"=w270, "Raw data"=w268, "File Name In"=w272, "DigCard"=i16 -1, "header"=w273, "Iter"=w271) -> ()  [unwired: 6 in]
              }
            }
            n99 = call "GPU_Process.vi"("DataFlag"=w244, "Ann Array Params"=w254, "Digitizer Settings"=w249, "Raw Data In"=w253) -> ("RF_Out"=w246:i16[][])  [unwired: 5 in, 2 out]
            n100 = Decrement(x=w248) -> (x-1=w250:i8)
            n101 = Power Of 2(x=w250) -> (2^x=w251:dbl)
            n102 = Decrement(x=w251) -> (x-1=w247:dbl)
            n103 = Absolute Value(x=w246) -> (abs(x)=w252:i16[][])
            n104 = for {
              tunnel: w252 -> [w266] mode=indexing
              tunnel: [w265] -> w245 mode=indexing
              tunnel: w247 -> [w264]
              n105 = call <vilib>:"Threshold Detector.vi"("threshold"=w264, "X"=w266) -> ("count"=w265:i32)  [unwired: 1 in, 2 out]
            }
          }
          frame True {
          }
        }
        n106 = Add Array Elements(numeric array=w224) -> (sum=w223:i32)
        n107 = Wait on Notification(notifier=w229, timeout in ms (-1)=5) -> (timed out?=w238:bool)  [unwired: 2 in, 3 out]
        n108 = Not(x=w238) -> (.not. x?=w237:bool)
        n109 = Bundle("gain"=w221, w220, "RF_Out"=w226, "count"=w223, w219) -> (w225:T21)  [unwired: 1 in]
        n110 = Lossy Enqueue Element(queue=w240, element=w225) -> ()  [unwired: 1 in, 4 out]
      }
      n111 = while {
        tunnel: w206 -> [w290]
        tunnel: w201 -> [w289]
        tunnel: [w288] -> w208
        tunnel: w216 -> [w279]
        tunnel: w215 -> [w287]
        tunnel: w186 -> [w286]
        tunnel: w198 -> [w285]
        tunnel: w192 -> [w284]
        tunnel: w190 -> [w283]
        tunnel: w185 -> [w281]
        tunnel: w202 -> [w280]
        tunnel: w185 -> [w277]
        tunnel: w197 -> [w276]
        tunnel: w189 -> [w275]
        tunnel: w183 -> [w274]
        i -> [w282]
        stop <- w278 stop-if-true
        # "Read queue and send to files. About same as reading channel by channel"
        n112 = stacked-sequence {
          seq-local: [w296 _ _ _ _] -> [_ w344 _ _ _]
          seq-local: [_ w338 _ _ _] -> [_ _ _ w486 _]
          tunnel: w290 -> [_ w347 _ _ _]
          tunnel: w289 -> [_ w346 _ _ _]
          tunnel: [_ w345 _ _ _] -> w288
          tunnel: w287 -> [w297 _ _ _ _]
          tunnel: w286 -> [_ w343 _ _ _]
          tunnel: w285 -> [w295 w342 _ w488 _]
          tunnel: w284 -> [_ w341 _ w485 _]
          tunnel: w283 -> [w294 w340 _ _ _]
          tunnel: w282 -> [w293 _ _ _ _]
          tunnel: w281 -> [w292 w339 _ w487 _]
          tunnel: w280 -> [_ w337 _ _ _]
          tunnel: w279 -> [_ _ w482 _ _]
          tunnel: [_ _ w481 _ _] -> w278
          tunnel: w277 -> [_ w336 _ _ _]
          tunnel: w276 -> [w291 w333 _ _ w522]
          tunnel: w275 -> [_ w335 _ _ _]
          tunnel: w274 -> [_ w334 _ _ _]
          frame #0 {
            # "Arm boards"
            n113 = case shown="\"AlazarTech\"" w295 {
              tunnel: w297 -> [w304 w324 w328]
              tunnel: [w303 w322 w327] -> w296
              tunnel: w294 -> [w302 _ w329]
              tunnel: w293 -> [_ _ _]
              tunnel: w292 -> [w298 w326 w331]
              tunnel: w291 -> [w299 w321 w330]
              frame "Acqiris Digitizer", Default {
                n114 = Unbundle By Name(w298) -> ("Digitizer ID Cluster.NI Instr Handles"=w301:refnum<k15>[])
                n115 = Reverse 1D Array(array=w301) -> (reversed array=w300:refnum<k15>[])
                n116 = for {
                  N -> [w309]
                  tunnel: w304 -> [w312]
                  tunnel: [w308] -> w303
                  tunnel: w302 -> [w307]
                  tunnel: w300 -> [w306] mode=indexing
                  tunnel: w299 -> [w305]
                  i -> [w310]
                  n117 = Subtract(x=w309, y=w310) -> (x-y=w311:i32)
                  n118 = case shown="1" w311 {
                    tunnel: [_ w320] -> w308
                    tunnel: w312 -> [_ w319]
                    tunnel: [w313 w318] -> _
                    tunnel: w306 -> [w314 w317]
                    tunnel: w307 -> [_ w316]
                    tunnel: w305 -> [_ w315]
                    frame 0, Default {
                      n119 = call <instrlib>:"niScope Initiate Acquisition.vi"("instrument handle"=w314) -> ("error out"=w313:errorcluster)  [unwired: 2 in, 12 out]
                    }
                    frame 1 {
                      # "Start Move"
                      n120 = call "Rapid Read_NI_Done.vi"("NI Card"=w317, "Motion Settings In"=w315, "records"=w316, "Pause?"=w319) -> ("Reverse?"=w320:bool, "error out"=w318:errorcluster)  [unwired: 10 in]
                    }
                  }
                }
              }
              frame "AlazarTech" {
                n121 = Unbundle By Name(w326) -> ("Digitizer ID Cluster.Acqiris/Alazar/SP ID"=w325:u32[])
                n122 = Index Array(array=w325) -> (element=w323:u32)  [unwired: 1 in]
                n123 = call "Rapid Read_Alazar_Done - ATS-SDK.vi"("Handle"=w323, "Motion Settings"=w321, "Pause?"=w324) -> ("Reverse?"=w322:bool)  [unwired: 10 in, 2 out]
              }
              frame "LeCroy" {
                n124 = Unbundle By Name(w331) -> ("Digitizer ID Cluster.LeCroy VISA"=w332:refnum<visa-resource-name>)
                n125 = call "Rapid Read_LeCroy_Done.vi"("Digitizer ID Cluster.LeCroy VISA"=w332, "Motion Settings In"=w330, "records"=w329, "Pause?"=w328) -> ("Reverse?"=w327:bool)  [unwired: 10 in, 1 out]
              }
            }
          }
          frame #1 {
            # "Read data"
            n126 = case shown="\"LeCroy\"" w342 {
              tunnel: w347 -> [w353 w419 w480]
              tunnel: w346 -> [w365 w429 _]
              tunnel: [w356 w422 w479] -> w345
              tunnel: w344 -> [w364 w428 w478]
              tunnel: w343 -> [w363 w427 _]
              tunnel: w341 -> [_ w413 w470]
              tunnel: w340 -> [w362 w426 _]
              tunnel: w339 -> [w361 _ _]
              tunnel: [_ _ w471] -> w338
              tunnel: w337 -> [_ _ w469]
              tunnel: w336 -> [w351 w417 w466]
              tunnel: w335 -> [_ _ _]
              tunnel: w334 -> [w350 w416 w472]
              tunnel: w333 -> [_ _ _]
              frame "Acqiris Digitizer", Default {
                n127 = Unbundle By Name(w361) -> ("NI ID/Channel"=w360:cluster{"NI ID":refnum<k15>, "NI CH":i32}[])
                n128 = for {
                  tunnel: w365 -> [w377]
                  tunnel: w364 -> [w371]
                  tunnel: w363 -> [w376] mode=indexing
                  tunnel: w362 -> [w375]
                  tunnel: w360 -> [w374] mode=indexing
                  tunnel: [w373] -> w349 mode=concatenating
                  tunnel: [w372] -> w359
                  tunnel: [w371] -> w358
                  tunnel: [w369] -> w357
                  tunnel: [w368] -> w355
                  tunnel: w351 -> [w367]
                  tunnel: w350 -> [w366]
                  i -> [w370]
                  n129 = case shown="True" w376 {
                    tunnel: w377 -> [_ w411]
                    tunnel: [_ w410] -> w372
                    tunnel: w370 -> [_ w404]
                    tunnel: [_ w400] -> w368
                    tunnel: w375 -> [_ w398]
                    tunnel: [FALSE ("status") w396] -> w369
                    tunnel: w374 -> [_ w394]
                    tunnel: [w386 w388] -> w373
                    tunnel: w367 -> [w384 w390]
                    tunnel: w366 -> [w381 w389]
                    frame False {
                      # "insert empty data if no receive channel"
                      n130 = Unbundle By Name(w381) -> ("Xmt/Rcv.XMIT"=w379:bool[])
                      n131 = Unbundle By Name(w384) -> ("rf points per line"=w383:i32, "lines per plane"=w382:i32)
                      n132 = Array Size(array=w379) -> (size(s)=w378:i32)
                      n133 = Compound Arithmetic op=MULTIPLY(w383, w382, w378) -> (w380:i32)
                      n134 = Initialize Array(i16 0, w380) -> (w386:i16[])
                    }
                    frame True {
                      n135 = Unbundle By Name(w394) -> ("NI CH"=w393:i32, "NI ID"=w395:refnum<k15>)
                      n136 = Equal To 0?(x=w404) -> (x = 0?=w403:bool)
                      n137 = property class="niScope"(reference=w395, "Fetch Record Number"=0, "Fetch Number of Records"=w398) -> (reference out=w406:refnum<k15>, error out=w405:errorcluster)  [unwired: 1 in]
                      n138 = Number To Decimal String(number=w393) -> (decimal integer string=w392:string)  [unwired: 1 in]
                      n139 = Select(t=1.0, s=w403, f=0.5) -> (s? t:f=w400:dbl)
                      n140 = call-poly <instrlib>:"niScope Fetch (poly).vi"("timeout"=w400, "error in"=w405, "numSamples"=w411, "channels"=w392, "instrument handle"=w406) -> ("error out"=w397:errorcluster, "wfm"=w391:i8[][], "wfm info"=w409:T22, "instrument handle out"=w399:refnum<k15>)  [unwired: 3 out]
                      n141 = call "DeInterleave.vi"("Digitizer Settings"=w390, "Ann Array Params"=w389, "Data in"=w391) -> ("Sorted Array Out"=w388:i16[])  [unwired: 8 in]
                      n142 = case shown="No Error" w397 {
                        tunnel: w399 -> [_ w412]
                        frame No Error {
                        }
                        frame Error {
                          n143 = call <instrlib>:"niScope Abort.vi"("instrument handle"=w412) -> ()  [unwired: 13 in, 2 out]
                        }
                      }
                      n144 = Index Array(array=w409) -> (element=w408:T23)  [unwired: 1 in]
                      n145 = Unbundle By Name(w397) -> ("status"=w396:bool)
                      n146 = Unbundle By Name(w408) -> ("gain"=w410:dbl)
                    }
                  }
                }
                n147 = expression code="x*1000"(w355) -> (w352:dbl)
                n148 = Bundle("gain"=w359, "Sorted Array Out"=w349, "Reverse?"=w358, "status"=w357, 0) -> (w354:T24)  [unwired: 1 in]
                n149 = Enqueue Element(queue=w353, element=w354, timeout in ms (-1)=w352) -> (queue out=w356:refnum<queue>)  [unwired: 1 in, 2 out]
              }
              frame "LeCroy" {
                n150 = for {
                  tunnel: w429 -> [w441]
                  tunnel: w428 -> [w436]
                  tunnel: w427 -> [w440] mode=indexing
                  tunnel: w426 -> [w439]
                  tunnel: [w438] -> w415 mode=concatenating
                  tunnel: [w437] -> w425
                  tunnel: [w436] -> w424
                  tunnel: [w434] -> w423
                  tunnel: [w433] -> w421
                  tunnel: w417 -> [w432]
                  tunnel: w416 -> [w431]
                  tunnel: w413 -> [w430]
                  i -> [w435]
                  n151 = case shown="True" w440 {
                    tunnel: w441 -> [_ _]
                    tunnel: [_ w453] -> w437
                    tunnel: w435 -> [_ w455]
                    tunnel: [_ w460] -> w433
                    tunnel: w439 -> [_ _]
                    tunnel: [FALSE ("status") FALSE ("status")] -> w434
                    tunnel: [w450 w458] -> w438
                    tunnel: w432 -> [w448 w456]
                    tunnel: w431 -> [w445 w459]
                    tunnel: w430 -> [_ _]
                    frame False {
                      # "insert empty data if no receive channel"
                      n152 = Unbundle By Name(w445) -> ("Xmt/Rcv.XMIT"=w443:bool[])
                      n153 = Unbundle By Name(w448) -> ("rf points per line"=w447:i32, "lines per plane"=w446:i32)
                      n154 = Array Size(array=w443) -> (size(s)=w442:i32)
                      n155 = Compound Arithmetic op=MULTIPLY(w447, w446, w442) -> (w444:i32)
                      n156 = Initialize Array(i16 0, w444) -> (w450:i16[])
                    }
                    frame True {
                      n157 = Equal To 0?(x=w455) -> (x = 0?=w463:bool)
                      n158 = call "GetAcqSeqLeCroy.vi"("Digitizer Settings"=w456, "Source (0: Channel 1)"=w455, "save?"=FALSE) -> ("Raw VGain (scale)"=w453:dbl, "Data Array"=w454:i16[][])  [unwired: 18 in, 5 out]
                      n159 = Select(t=1.0, s=w463, f=0.5) -> (s? t:f=w460:dbl)
                      n160 = call "DeInterleave.vi"("Digitizer Settings"=w456, "Ann Array Params"=w459, "Data in"=w454) -> ("Sorted Array Out"=w458:i16[])  [unwired: 8 in]
                    }
                  }
                }
                n161 = expression code="x*1000"(w421) -> (w418:dbl)
                n162 = Bundle("Raw VGain (scale)"=w425, "Sorted Array Out"=w415, "Reverse?"=w424, "status"=w423, 0) -> (w420:T25)  [unwired: 1 in]
                n163 = Enqueue Element(queue=w419, element=w420, timeout in ms (-1)=w418) -> (queue out=w422:refnum<queue>)  [unwired: 1 in, 2 out]
              }
              frame "AlazarTech" {
                n164 = Bundle By Name(cluster=w466, "DigTimeOut"=400.0 ("time out")) -> (w465:T8)
                n165 = call "AlazarStackChannels1Pass.vi"("AlazarCluster"=w470, "Digitizer Settings"=w465, "Extra Shift"=w469, "Ann Array Params"=w472) -> ("Voltage Scale"=w468:dbl, "Return Code"=w471:u32, "DataInterleavedOut"=w467:i16[])  [unwired: 3 in, 2 out]
                n166 = Equal?(x=w471, y=u32 579) -> (x = y?=w476:bool)
                n167 = Bundle("Voltage Scale"=w468, "DataInterleavedOut"=w467, "Reverse?"=w478, w476, 1) -> (w474:T26)  [unwired: 1 in]
                n168 = Enqueue Element(queue=w480, element=w474, timeout in ms (-1)=20.0 ("time out")) -> (queue out=w479:refnum<queue>)  [unwired: 1 in, 2 out]
              }
            }
          }
          frame #2 {
            n169 = Wait on Notification(notifier=w482, timeout in ms (-1)=5) -> (timed out?=w483:bool)  [unwired: 2 in, 3 out]
            n170 = Not(x=w483) -> (.not. x?=w481:bool)
          }
          frame #3 {
            n171 = case shown="\"AlazarTech\"" w488 {
              tunnel: w485 -> [_ w491]
              tunnel: w487 -> [_ w490]
              tunnel: w486 -> [_ w489]
              frame "Acqiris Digitizer", Default {
              }
              frame "AlazarTech" {
                n172 = case shown="512, Default" w489 {
                  tunnel: w491 -> [_ w505]
                  tunnel: w490 -> [_ w504]
                  frame 0 {
                  }
                  frame 512, Default {
                    w496 = u32 268435538 items=["Data Width"=268435465, "Set/Get Async BuffSize"=268435513, "Set/Get Async Buffcount"=268435520, "Get Data Format"=268435522, "Get Samples Per Timestamp Clock"=268435524, "Get Records Captured"=268435525, "Get Async Buffers Pending"=268435536, "Get Async Buffers Pending Full"=268435537, "Get Async Buffers Pending Empty"=268435538, "ECC Mode"=268435528, "Get Aux Input Level"=268435529, "Get Channels Per Board"=268435568, "Pack Mode"=268435570, "Get FPGA Temperature"=268435584] ("Parameter")
                    w497 = u32 268435537 items=["Data Width"=268435465, "Set/Get Async BuffSize"=268435513, "Set/Get Async Buffcount"=268435520, "Get Data Format"=268435522, "Get Samples Per Timestamp Clock"=268435524, "Get Records Captured"=268435525, "Get Async Buffers Pending"=268435536, "Get Async Buffers Pending Full"=268435537, "Get Async Buffers Pending Empty"=268435538, "ECC Mode"=268435528, "Get Aux Input Level"=268435529, "Get Channels Per Board"=268435568, "Pack Mode"=268435570, "Get FPGA Temperature"=268435584] ("Parameter")
                    w502 = u32 268435536 items=["Data Width"=268435465, "Set/Get Async BuffSize"=268435513, "Set/Get Async Buffcount"=268435520, "Get Data Format"=268435522, "Get Samples Per Timestamp Clock"=268435524, "Get Records Captured"=268435525, "Get Async Buffers Pending"=268435536, "Get Async Buffers Pending Full"=268435537, "Get Async Buffers Pending Empty"=268435538, "ECC Mode"=268435528, "Get Aux Input Level"=268435529, "Get Channels Per Board"=268435568, "Pack Mode"=268435570, "Get FPGA Temperature"=268435584] ("Parameter")
                    n173 = Unbundle By Name(w504) -> ("Digitizer ID Cluster.Acqiris/Alazar/SP ID"=w503:u32[])
                    n174 = Index Array(array=w503) -> (element=w495:u32)  [unwired: 1 in]
                    n175 = call "AlazarGetParameter.vi"("Parameter"=w502, "Handle"=w495) -> ("error out"=w499:errorcluster, "Handle"=w501:u64)  [unwired: 2 in, 2 out]
                    n176 = call "AlazarGetParameter.vi"("error in (no error)"=w499, "Parameter"=w496, "Handle"=w501) -> ("error out"=w498:errorcluster, "Handle"=w500:u64)  [unwired: 1 in, 2 out]
                    n177 = call "AlazarGetParameter.vi"("error in (no error)"=w498, "Parameter"=w497, "Handle"=w500) -> ("error out"=w494:errorcluster, "Value"=w492:i32, "Handle"=w493:u64)  [unwired: 1 in, 1 out]
                    n178 = case shown="2, Default" w492 {
                      selector: w492 -> [_ w510]
                      tunnel: w505 -> [_ w512]
                      tunnel: w494 -> [_ w507]
                      tunnel: w493 -> [_ w506]
                      frame 0, 1 {
                      }
                      frame 2, Default {
                        # "Delete surplus buffers"
                        n179 = Decrement(x=w510) -> (x-1=w508:i32)
                        n180 = Unbundle(w512) -> ("data value reference"=w511:refnum<data-value>)  [unwired: 2 out]
                        n181 = for {
                          N: w508 -> [_]
                          tunnel: w511 -> [w515]
                          tunnel: u32 1 ("uTimeout_ms") -> [w516]
                          tunnel: w507 -> [w514]
                          tunnel: w506 -> [w513]
                          n182 = in-place {
                            in-place-border: w516 -> [w521]
                            in-place-border: w514 -> [w518]
                            in-place-border: w513 -> [w517]
                            n183 = in-place-dvr #1(w515) -> (w520:u16[])  [unwired: 1 out]
                            n184 = call "AlazarWaitNextAsyncBufferCompleteU16.vi"("error in (no error)"=w518, "Timeout (ms)"=w521, "Buffer"=w520, "Handle"=w517) -> ("Buffer"=w519:u16[])  [unwired: 3 out]
                            n185 = in-place-dvr #1(w519) -> ()  [unwired: 2 out]
                          }
                        }
                      }
                    }
                  }
                }
              }
            }
          }
          frame #4 {
            # "Check if motion program is paused at end of run. Rare case of done may come up."
            n186 = case shown="4" 0 {
              tunnel: w522 -> [_ w526]
              frame 0, Default {
              }
              frame 4 {
                n187 = Unbundle By Name(w526) -> ("Motion Bd ID"=w525:u8, "Motion System"=w524:T5)
                n188 = case shown="\"NI 735x\"" w524 {
                  tunnel: w525 -> [_ w527]
                  frame "MM3000", Default {
                  }
                  frame "NI 735x" {
                    n189 = disable-structure shown="Disabled" {
                      disable-tunnel: w527 -> [w528 _]
                      frame Disabled {
                        n190 = while {
                          tunnel: [w540] -> _
                          tunnel: [w536] -> _
                          tunnel: enum16{"Done", "Playing", "Paused", "Storing"}."Paused" ("Program Status") -> [w539]
                          tunnel: w528 -> [w538]
                          tunnel: [w532] -> _
                          tunnel: [30 ("DeviceIn")] -> w529
                          i -> [w532]
                          stop <- w533 stop-if-true
                          n191 = call <vilib>:"Read Program Status.flx"("Program (1)"=T19 8, "Board Id"=w538) -> ("error out"=w536:errorcluster, "Bd Id Out"=w540:T27, "Program Status"=w537:enum16{"Done", "Playing", "Paused", "Storing"})  [unwired: 4 in, 1 out]
                          n192 = Unbundle(w536) -> ("status"=w535:bool)  [unwired: 2 out]
                          n193 = Equal?(x=w539, y=w537) -> (x = y?=w534:bool)
                          n194 = Or(x=w534, y=w535) -> (x .or. y?=w533:bool)
                        }
                        n195 = Wait (ms)(milliseconds to wait=w529) -> ()  [unwired: 1 out]
                      }
                      frame Enabled {
                      }
                    }
                  }
                }
              }
            }
          }
        }
      }
      n196 = Release Queue(queue=w208, force destroy? (F)=w204) -> ()  [unwired: 1 in, 3 out]
    }
    frame #5 {
      n197 = Unbundle By Name(w542) -> ("Motion System"=w544:T5)
      n198 = Unbundle By Name(w547) -> ("Main Digitizer"=w546:T9, "Dig Config"=w545:T10)
      n199 = case shown="\"NI 735x\"" w544 {
        tunnel: w549 -> [w554 _]
        tunnel: w542 -> [w553 _]
        frame "NI 735x" {
          n200 = disable-structure shown="Disabled" {
            disable-tunnel: w554 -> [w557 _]
            disable-tunnel: w553 -> [w556 _]
            frame Disabled {
              n201 = Unbundle By Name(w556) -> ("Motion Bd ID"=w555:u8)
              n202 = call <vilib>:"Enable Breakpoint Output.flx"("Enable Breakpoint"=FALSE, "Axis or Encoder"=w557, "Board ID"=w555) -> ()  [unwired: 1 in, 6 out]
            }
            frame Enabled {
            }
          }
        }
        frame "No Motion Card", Default {
        }
      }
      n203 = case shown="\"AlazarTech\"" w546 {
        tunnel: w547 -> [w560 w565 _]
        tunnel: w548 -> [_ w563 _]
        frame "Acqiris Digitizer" {
          n204 = Unbundle By Name(w560) -> ("Digitizer ID Cluster.NI Instr Handles"=w559:refnum<k15>[])
          n205 = for {
            tunnel: w559 -> [w561] mode=indexing
            n206 = call <instrlib>:"niScope Abort.vi"("instrument handle"=w561) -> ()  [unwired: 13 in, 2 out]
          }
        }
        frame "AlazarTech" {
          n207 = Unbundle By Name(w565) -> ("Digitizer ID Cluster.Acqiris/Alazar/SP ID"=w564:u32[])
          n208 = Unbundle By Name(w563) -> ("data value reference"=w562:refnum<data-value>)
          n209 = for {
            tunnel: w564 -> [w567] mode=indexing
            n210 = call "AlazarAbortAsyncRead.vi"("Handle"=w567) -> ("Handle"=w569:u64, "error out"=w568:errorcluster)  [unwired: 1 in, 1 out]
            n211 = call "AlazarConfigureAuxIO.vi"("error in (no error)"=w568, "Mode"=u32 13, "Handle"=w569) -> ()  [unwired: 1 in, 3 out]
          }
          n212 = Delete Data Value Reference(data value reference=w562) -> ()  [unwired: 1 in, 2 out]
        }
        frame "LeCroy", Default {
        }
      }
      n213 = Cancel Notification(0:w550) -> ()  [unwired: 1 in, 3 out]
      n214 = case shown="\"Hawaii\", Default" w551 {
        tunnel: w542 -> [w575 _]
        frame "Hawaii", Default {
          w576 = u16 1 items=["Function Gen Input", "Motion Trig", "Internal RT Motion Trig", "Internal CTR 1 Output"] ("Trig Source")
          n215 = Unbundle By Name(w575) -> ("GL Ref Out"=w574:refnum<k7>)
          n216 = call "RouteTrigSource.vi"("Galil.IGalil"=w574, "Trig Source"=w576) -> ()  [unwired: 9 in, 1 out]
        }
        frame "UHI Allen", "CUMC RT" {
        }
      }
      n217 = case shown="\"5-CH pulser w/ ann array\"" w545 {
        tunnel: w552 -> [_ w570]
        frame "Single channel", Default {
        }
        frame "5-CH pulser w/ ann array" {
          n218 = for {
            tunnel: w570 -> [w573] mode=indexing
            n219 = call <vilib>:"DAQmx Stop Task.vi"("task/channels in"=w573) -> ("task out"=w572:refnum<k21>, "error out"=w571:errorcluster)  [unwired: 13 in]
            n220 = call <vilib>:"DAQmx Clear Task.vi"("task in"=w572, "error in"=w571) -> ()  [unwired: 13 in, 1 out]
          }
        }
      }
      n221 = Unbundle By Name(w542) -> ("Motion System"=w543:T5)
    }
  }
  n222 = case shown="\"NI 735x\"" w6 {
    tunnel: w26 -> [w578 w611 _]
    tunnel: w25 -> [w581 _ _]
    tunnel: w24 -> [w580 w605 _]
    tunnel: w23 -> [w579 w612 _]
    tunnel: w5 -> [w577 w613 _]
    frame "NI 735x" {
      n223 = disable-structure shown="Disabled" {
        disable-tunnel: w581 -> [w604 _]
        disable-tunnel: w580 -> [w603 _]
        disable-tunnel: w579 -> [w602 _]
        disable-tunnel: w578 -> [w587 _]
        disable-tunnel: w577 -> [w583 _]
        frame Disabled {
          # "Return to start location and reset to original value"
          n224 = Unbundle By Name(w583) -> ("Motor Parameters.velocity ct/s"=w589:dbl[], "Motor Parameters.accel ct/s^2"=w588:dbl[], "Motion Bd ID"=w582:u8)
          n225 = call-poly <vilib>:"Wait for Move Complete.flx"("error in (no error)"=w603, "Board ID"=w582) -> ("error out"=w590:errorcluster, "Bd ID Out"=w591:T27)  [unwired: 6 in, 2 out]
          n226 = call <vilib>:"Stop Program.flx"("error in (no error)"=w590, "Program (1)"=w604, "Board ID"=w591) -> ("error out"=w599:errorcluster, "Bd ID Out"=w600:T27)  [unwired: 4 out]
          n227 = Decrement(x=w587) -> (x-1=w586:u16)
          n228 = call "MoveMotor.vi"("error in (no error)"=w599, "Target Position (0)"=w602, "Axis or Vector Space"=w587, "Motion Bd ID"=w600) -> ("error out"=w593:errorcluster, "Resource Output"=w592:u16, "Bd ID Out"=w594:u8)  [unwired: 5 in]
          n229 = Index Array(array=w589, index=w586) -> (element=w585:dbl)
          n230 = Index Array(array=w588, index=w586) -> (element=w584:dbl)
          n231 = call "Load Acceleration/Deceleration.flx"("Acceleration (100000)"=w584, "error in (no error)"=w593, "Axis or Vector Space"=w592, "Board ID"=w594) -> ("error out"=w597:errorcluster, "Resource Output"=w595:T28, "Bd ID Out"=w596:T27)  [unwired: 1 in, 2 out]
          n232 = call <vilib>:"Load Velocity.flx"("Velocity (10000)"=w585, "error in (no error)"=w597, "Axis or Vector Space"=w595, "Board ID"=w596) -> ("error out"=→"error out":errorcluster, "Bd ID Out"=→"Bd ID Out":T27)  [unwired: 4 out]
        }
        frame Enabled {
        }
      }
    }
    frame "Galil" {
      (unwired) Command_Menu."Halt Execute" ("Command")
      n233 = Unbundle By Name(w613) -> ("Motor Parameters.velocity ct/s"=w637:dbl[], "Motor Parameters.accel ct/s^2"=w636:dbl[], "GL Ref Out"=w606:refnum<k7>)
      n234 = call "GL Command Set.vi"("error in (no error)"=w605, "Value"=-1, "Galil.IGalil"=w606) -> ("error out"=w608:errorcluster, "ref out"=w607:refnum<k7>)  [unwired: 4 in, 3 out]
      n235 = Decrement(x=w611) -> (x-1=w617:u16)
      n236 = call "GL Command Set.vi"("Command"=Command_Menu."BreakPoint", "error in (no error)"=w608, "Value"=0, "Axis"=w617, "Galil.IGalil"=w607) -> ("error out"=w622:errorcluster, "Axis Out"=w618:T29, "ref out"=w623:refnum<k7>)  [unwired: 2 in, 2 out]
      n237 = call "GL CheckForMotion.vi"("error in"=w622, "Axis"=w618, "Refnum in"=w623) -> ("error out"=w620:errorcluster, "Axis out"=w619:T29, "Refnum out"=w621:refnum<k7>)  [unwired: 6 in]
      n238 = Index Array(array=w637, index=w617) -> (element=w627:dbl)
      n239 = Index Array(array=w636, index=w617) -> (element=w626:dbl)
      n240 = call "GL Set Operation Mode.vi"("position cts (abs/rel)"=w612, "error in (no error)"=w620, "Axis"=w619, "Galil.IGalil"=w621) -> ("error out"=w614:errorcluster, "Axis Out Output"=w625:T29, "Galil Out"=w624:refnum<k7>)  [unwired: 5 in]
      n241 = call "GL Command Set.vi"("Command"=Command_Menu."Velocity", "error in (no error)"=w614, "Value"=w627, "Axis"=w625, "Galil.IGalil"=w624) -> ("error out"=w634:errorcluster, "Axis Out"=w631:T29, "ref out"=w635:refnum<k7>)  [unwired: 2 in, 2 out]
      n242 = call "GL Command Set.vi"("Command"=Command_Menu."Acceleration", "error in (no error)"=w634, "Value"=w626, "Axis"=w631, "Galil.IGalil"=w635) -> ("error out"=w632:errorcluster, "Axis Out"=w630:T29, "ref out"=w633:refnum<k7>)  [unwired: 2 in, 2 out]
      n243 = call "GL Command Set.vi"("Command"=Command_Menu."Deceleration", "error in (no error)"=w632, "Value"=w626, "Axis"=w630, "Galil.IGalil"=w633) -> ()  [unwired: 2 in, 5 out]
    }
    frame "No Motion Card", Default {
    }
  }
